vi "UHR-Fleezers Control (host) - 12.1.vi"() -> ()   [LabVIEW 2012] (continued)
            n1097 = Divide(x=w2495, y=w2493) -> (x/y=w2492:dbl[])
            n1098 = Divide(x=w2542, y=w2540) -> (x/y=w2526:dbl[])
            n1099 = Divide(x=w2541, y=w2540) -> (x/y=w2525:dbl[])
            n1100 = Divide(x=w2539, y=w2537) -> (x/y=w2524:dbl[])
            n1101 = Divide(x=w2538, y=w2537) -> (x/y=w2523:dbl[])
            n1102 = Divide(x=w2509, y=w2493) -> (x/y=w2508:dbl[])
            n1103 = Divide(x=w2507, y=w2491) -> (x/y=w2506:dbl[])
            n1104 = Build Array(w2526, w2525, w2540, w2524, w2523, w2537, w2492, w2508, w2493, w2490, w2506, w2491, w2504, w2503) -> (w2502:dbl[][])
            n1105 = Bundle("T1 Y", "T1 X", "T1 Sum", "T2 Y", "T2 X", "T2 Sum", "T1 FB Y", "T1 FB X", "T1 FB Sum", "T2 FB Y", "T2 FB X", "T2 FB Sum", "PSD X", "PSD Y Sum") -> (w2489:T39)  [unwired: 1 out]
            n1106 = To Word Integer(number=w2544) -> (16bit integer=w2488:i16[])
            n1107 = Cluster To Array(cluster=w2489) -> (array=w2535:string[])
          }
        }
      }
    }
    "AI labels" <- w1629
    n1108 = Decimate 1D Array(w1603) -> (w1627:u32[], w1571:u32[])
    n1109 = local read "DMA Update Period (s)"() -> (w1639:dbl)
    n1110 = Build Array(w1627, w1571) -> (w1697:u32[][])
    n1111 = local read "Data Period (s)"() -> (w1477:dbl)
    n1112 = local read "BD 1 Frequency 2 (MHz)"() -> (w1510:dbl)
    n1113 = local read "BD 1 Frequency 1 (MHz)"() -> (w1511:dbl)
    n1114 = Decimate 1D Array(w1518) -> (w1542:i16[], w1541:i16[], w1539:i16[], w1538:i16[])  [unwired: 9 out]
    n1115 = To Double Precision Float(number=w1697) -> (double precision float=w1698:dbl[][])
    n1116 = local read "APD Integration Time (s)"() -> (w1584:dbl)
    n1117 = Multiply(x=w1477, y="Trap Pos. Disp. Downsample") -> (x*y=w1475:dbl)
    n1118 = Divide(x=w1542, y=w1541) -> (x/y=w1543:dbl[])
    n1119 = Divide(x=w1539, y=w1538) -> (x/y=w1540:dbl[])
    n1120 = feedback #6(0.0) -> (w1556:dbl)
    n1121 = Add(x=w1639, y=w1556) -> (x+y=w1737:dbl)
    n1122 = feedback-in #6(w1737) -> ()
    n1123 = local read "AOM X Cal (nm/MHz)"() -> (w1508:dbl)
    n1124 = To Time Stamp(1:w1556) -> (0:w1555:timestamp)
    n1125 = Split 1D Array(array=w1543, index="N El. to Ave.") -> (second subarray=w1546:dbl[])  [unwired: 1 out]
    n1126 = Split 1D Array(array=w1540, index="N El. to Ave.") -> (second subarray=w1545:dbl[])  [unwired: 1 out]
    n1127 = Multiply(x=w1477, y="Trap Disp. Downsample") -> (x*y=w1557:dbl)
    "Display Period (s)" <- w1557
    n1128 = for "Trap AI" {
      tunnel: [w2287] -> w1731 mode=indexing
      tunnel: w1555 -> [w2277]
      tunnel: "Trap Disp. Downsample" -> [w2285]
      tunnel: w1630 -> [w2283] mode=indexing
      tunnel: w1477 -> [w2282]
      tunnel: w1629 -> [w2281] mode=indexing
      tunnel: w1554 -> [w2280]
      tunnel: [w2279] -> w1595 mode=indexing
      tunnel: w1557 -> [w2278]
      workers-P: _ -> [_]
      n1129 = Bundle By Name("Y"=w2283, "dt"=w2282) -> (w2284:waveform(dbl))  [unwired: 1 out]
      n1130 = Set Waveform Attribute(5:w2281, 6:w2280, 7:w2284) -> (3:w2279:waveform(dbl))  [unwired: 1 in, 2 out]
      n1131 = call "downsample 1D array - double.vi"("Ave N"=w2285, "Array In"=w2283) -> ("Array Out"=w2286:dbl[])  [unwired: 1 out]
      n1132 = Bundle By Name(cluster=w2279, "t0"=w2277, "Y"=w2286, "dt"=w2278) -> (w2287:waveform(dbl))
    }
    n1133 = Bundle("BD 1 Frequency 1 (MHz)"=w1511, "BD 1 Frequency 2 (MHz)"=w1510) -> (w1512:T40)  [unwired: 1 out]
    n1134 = call-poly <vilib>:"Mean.vi"("X"=w1545) -> ("mean"=w1533:dbl)  [unwired: 1 out]
    n1135 = call-poly <vilib>:"Mean.vi"("X"=w1546) -> ("mean"=w1534:dbl)  [unwired: 1 out]
    n1136 = Reciprocal(x=w1557) -> (1/x=→"Trap Disp. Freq. (Hz)":dbl)
    n1137 = Cluster To Array(cluster=w1512) -> (array=w1509:dbl[])
    n1138 = local read "Trap X AI1 (DMA)"() -> (w1544:T13)
    n1139 = local read "Data points/scans (MCL)"() -> (w1709:dbl)
    n1140 = To Fixed-Point(number=w1533) -> (fixed-point=w1531:fxp<+/-,16,1>)  [unwired: 1 in]
    n1141 = To Fixed-Point(number=w1534) -> (fixed-point=w1532:fxp<+/-,16,1>)  [unwired: 1 in]
    n1142 = Bundle("Trap 1 Pos.", "Trap 2 Pos.") -> (w1553:cluster{string, string})  [unwired: 1 out]
    n1143 = Bundle By Name(cluster=w1544, "Set 1"=w1532, "Set 2"=w1531) -> (→"Trap X AI1 (DMA)":T13)
    n1144 = Cluster To Array(cluster=w1553) -> (array=w1550:string[])
    n1145 = Bundle("APD 1", "APD 2") -> (w1730:cluster{string, string})  [unwired: 1 out]
    n1146 = Select(t=-1.0, s="Negate Y Axis", f=1.0) -> (s? t:f=w1494:dbl)
    n1147 = for "Trap Position" {
      tunnel: w1559 -> [w1926] mode=indexing
      tunnel: "Trap Pos. Disp. Downsample" -> [w1925]
      tunnel: w1475 -> [w1923]
      tunnel: w1555 -> [w1922]
      tunnel: w1554 -> [w1920]
      tunnel: w1550 -> [w1919] mode=indexing
      tunnel: [w1918] -> w1464 mode=indexing
      tunnel: w1509 -> [w1916] mode=indexing
      tunnel: w1508 -> [w1914]
      tunnel: w1494 -> [w1913]
      n1148 = call "downsample 1D array - double.vi"("Ave N"=w1925, "Array In"=w1926) -> ("Array Out"=w1924:dbl[])  [unwired: 1 out]
      n1149 = Subtract(x=w1924, y=w1916) -> (x-y=w1917:dbl[])
      n1150 = Multiply(x=w1914, y=w1917) -> (x*y=w1915:dbl[])
      n1151 = Multiply(x=w1913, y=w1915) -> (x*y=w1912:dbl[])
      n1152 = Bundle By Name("Y"=w1912, "dt"=w1923, "t0"=w1922) -> (w1921:waveform(dbl))  [unwired: 1 out]
      n1153 = Set Waveform Attribute(5:w1919, 6:w1920, 7:w1921) -> (3:w1918:waveform(dbl))  [unwired: 1 in, 2 out]
    }
    n1154 = Cluster To Array(cluster=w1730) -> (array=w1727:string[])
    n1155 = for "APD" {
      tunnel: w1698 -> [w2266] mode=indexing
      tunnel: w1584 -> [w2274]
      tunnel: [w2270] -> w1591 mode=indexing
      tunnel: "APD Disp. Scale" -> [w2271]
      tunnel: w1554 -> [w2269]
      tunnel: w1727 -> [w2268] mode=indexing
      tunnel: "APD Disp. Downsample" -> [w2264]
      tunnel: [w2267] -> w1726
      workers-P: _ -> [_]
      tunnel: w1555 -> [w2263]
      n1156 = call "integrate 1D array interval - double.vi"("Ave N"=w2264, "Array In"=w2266) -> ("Array Out"=w2265:dbl[])  [unwired: 1 out]
      n1157 = Multiply(x=w2274, y=w2264) -> (x*y=w2267:dbl)
      n1158 = Divide(x=w2265, y=w2271) -> (x/y=w2272:dbl[])
      n1159 = Bundle By Name("t0"=w2263, "Y"=w2272, "dt"=w2267) -> (w2273:waveform(dbl))  [unwired: 1 out]
      n1160 = Set Waveform Attribute(5:w2268, 6:w2269, 7:w2273) -> (3:w2270:waveform(dbl))  [unwired: 1 in, 2 out]
    }
    "APD Display Period (s)" <- w1726
    n1161 = Reciprocal(x=w1726) -> (1/x=→"APD Display Freq. (Hz)":dbl)
    n1162 = local read "Display Period (s)"() -> (w1615:dbl)
    n1163 = Increment(x=w1709) -> (x+1=w1710:dbl)
    n1164 = To Double Precision Float(number=w1627) -> (double precision float=w1626:dbl[])
    n1165 = Index Array(array=w1464, index=0) -> (element=w1468:waveform(dbl))
    n1166 = Index Array(array=w1464, index=1) -> (element=w1463:waveform(dbl))
    n1167 = feedback #7(w1710) -> (w1713:dbl)
    n1168 = Select(t=0, s=w1700, f=w1713) -> (s? t:f=w1706:dbl)
    n1169 = Array Size(array=w1626) -> (size(s)=w1712:i32)
    n1170 = Add(x=w1712, y=w1706) -> (x+y=w1707:dbl)
    n1171 = Unbundle By Name(w1468) -> ("Y"=w1469:dbl[])
    n1172 = feedback #8(w1627) -> (w1696:u32[])
    n1173 = Build Array (concatenate)(w1696, w1627) -> (w1693:u32[])
    n1174 = feedback #9(w1571) -> (w1590:u32[])
    n1175 = Divide(x="Bead Sep. Int. Time (s)", y=w1615) -> (x/y=w1504:dbl)
    n1176 = Build Array (concatenate)(w1590, w1571) -> (w1589:u32[])
    n1177 = Add(x=w1469, y="FB Trap Pos Offset") -> (x+y=w1467:dbl[])
    "T1 x pos data" <- w1467
    n1178 = Greater?(x=w1707, y=w1709) -> (0:w1708:bool)
    n1179 = feedback #10(w1467) -> (w1506:dbl[])
    n1180 = Build Array (concatenate)(w1467, w1506) -> (w1505:dbl[])
    n1181 = Bundle By Name(cluster=w1468, "Y"=w1467) -> (w1466:waveform(dbl))
    n1182 = Select(t=w1706, s=w1708, f=w1707) -> (s? t:f=w1705:dbl)
    n1183 = feedback-in #7(w1705) -> ()
    n1184 = Array Size(array=w1693) -> (size(s)=w1690:i32)
    n1185 = Array Size(array=w1627) -> (size(s)=w1692:i32)
    n1186 = local read "MCL Scanning"() -> (w1703:bool)
    n1187 = local read "APD Integration Time (s)"() -> (w1598:dbl)
    n1188 = Bundle(w1466, w1463) -> (w1462:cluster{waveform(dbl), waveform(dbl)})  [unwired: 1 out]
    n1189 = Build Array (concatenate)(w1591, w1731) -> (w1593:waveform(dbl)[])
    "All Signals" <- w1593
    n1190 = Split 1D Array(array=w1505, index=w1504) -> (first subarray=w1498:dbl[])  [unwired: 1 out]
    n1191 = feedback-in #10(w1498) -> ()
    n1192 = Multiply(x=w1692, y="APD Ave N") -> (x*y=w1691:dbl)
    n1193 = Greater?(x=w1690, y=w1691) -> (0:w1694:bool)
    n1194 = Not(x=w1708) -> (.not. x?=w1702:bool)
    n1195 = Cluster To Array(cluster=w1462) -> (array=w1438:waveform(dbl)[])
    "Trap Positions" <- w1438
    n1196 = To Double Precision Float(number=w1571) -> (double precision float=w1570:dbl[])
    n1197 = call-poly <vilib>:"Mean.vi"("X"=w1498) -> ("mean"=w1497:dbl)  [unwired: 1 out]
    "Mean T1 Position (nm)" <- w1497
    n1198 = Subtract(x=w1498, y=w1497) -> (x-y=w1503:dbl[])
    n1199 = Square(x=w1503) -> (x^2=w1502:dbl[])
    n1200 = And(x=w1702, y=w1703) -> (x .and. y?=w1704:bool)
    n1201 = call-poly <vilib>:"Mean.vi"("X"=w1502) -> ("mean"=w1501:dbl)  [unwired: 1 out]
    n1202 = case shown="True" w1694 {
      tunnel: w1693 -> [w2046 w2053]
      tunnel: [w2046 w2051] -> w1644
      tunnel: w1691 -> [_ w2048]
      tunnel: w1690 -> [_ w2052]
      tunnel: w1589 -> [w2045 w2050]
      tunnel: [w2045 w2047] -> w1586
      frame False {
      }
      frame True {
        n1203 = Subtract(x=w2052, y=w2048) -> (x-y=w2049:dbl)
        n1204 = Array Subset(array=w2053, index=w2049, length=w2048) -> (w2051:u32[])
        n1205 = Array Subset(array=w2050, index=w2049, length=w2048) -> (w2047:u32[])
      }
    }
    n1206 = feedback-in #8(w1644) -> ()
    n1207 = feedback-in #9(w1586) -> ()
    n1208 = Square Root(x=w1501) -> (sqrt(x)=w1500:dbl)
    n1209 = Or(x=w1704, y=w1700) -> (x .or. y?=w1701:bool)
    n1210 = Equal?(x="Tab Control 6", y=T28."High Res Display") -> (x = y?=w1633:bool)
    n1211 = Multiply(x="APD Disp. Scale", y=w1591) -> (x*y=w1600:waveform(dbl)[])
    n1212 = Multiply(x=10.0, y=w1500) -> (x*y=→"Trap 1 Position RMS (A)":dbl)
    n1213 = Multiply(x="APD Disp. Downsample", y=w1598) -> (x*y=w1596:dbl)
    n1214 = Divide(x=w1600, y=w1596) -> (x/y=w1568:waveform(dbl)[])
    n1215 = case "For displaying the high resolution display (no downsampling)" shown="True" w1633 {
      tunnel: w1595 -> [_ w1946]
      frame False {
      }
      frame True {
        n1216 = Index Array(array=w1946, index="High Res. Display") -> (element=w1947:waveform(dbl))
        n1217 = call <vilib>:"Std Deviation and Variance.vi"("X"=w1947) -> ("mean"=w1954:dbl, "standard deviation"=w1959:dbl)  [unwired: 1 in, 1 out]
        "Mean Intensity" <- w1954
        "Sigma" <- w1959
        n1218 = Subtract(x=w1947, y=w1954) -> (x-y=w1953:waveform(dbl))
        n1219 = Select(t=w1953, s="Subtract mean", f=w1947) -> (s? t:f=→"1 Channel":waveform(dbl))
        n1220 = Divide(x=w1959, y=w1954) -> (x/y=→"Sigma/Mean":dbl)
        n1221 = feedback #11(1) -> (w1948:i32)
        n1222 = Greater Or Equal?(x=w1948, y="Slow mean N ave.") -> (x >= y?=w1961:bool)
        n1223 = Increment(x=w1948) -> (x+1=w1963:i32)
        n1224 = Select(t=1, s=w1961, f=w1963) -> (s? t:f=w1950:i32)
        n1225 = feedback-in #11(w1950) -> ()
        n1226 = feedback #12() -> (w1951:waveform(dbl))  [unwired: 1 out]
        n1227 = case shown="Default" w1948 {
          tunnel: [w1966 w1969] -> w1952
          tunnel: w1951 -> [w1968 _]
          tunnel: w1947 -> [w1967 w1969]
          frame Default {
            n1228 = call-poly <vilib>:"Append Waveforms.vi"("waveform B"=w1967, "waveform A"=w1968) -> ("waveform out"=w1966:waveform(dbl))  [unwired: 1 in, 8 out]
          }
          frame 1 {
          }
        }
        n1229 = feedback-in #12(w1952) -> ()
        n1230 = case shown="True" w1961 {
          tunnel: w1952 -> [_ w1965]
          frame False {
          }
          frame True {
            n1231 = call-poly <vilib>:"Mean.vi"("X"=w1965) -> ("mean"=→"Slow mean":dbl)  [unwired: 1 out]
          }
        }
      }
    }
    n1232 = Index Array(array=w1568, index=0) -> (element=w1578:waveform(dbl))
    n1233 = Index Array(array=w1568, index=1) -> (element=w1576:waveform(dbl))
    n1234 = case "For computing FFTs for display" shown="True" "Compute FFT" {
      tunnel: w1595 -> [_ w2660]
      frame False {
      }
      frame True {
        n1235 = Build Array("FFT 1 Choice 1", "FFT 1 Choice 2", "FFT 2 Choice 1", "FFT 2 Choice 2") -> (w2653:u16[])
        n1236 = Array Size(array=w2660) -> (size(s)=w2659:i32)
        n1237 = feedback-in #13(w2653) -> ()
        n1238 = feedback #13(u16[] [100, 100, 100, 100]) -> (w2654:u16[])
        n1239 = feedback-in #14("# Spectra to Ave.") -> ()
        n1240 = feedback #14("# Spectra to Ave.") -> (w2651:dbl)
        n1241 = Not Equal?(x="# Spectra to Ave.", y=w2651) -> (x != y?=w2650:bool)
        n1242 = Not Equal?(x=w2653, y=w2654) -> (x != y?=w2652:bool)
        n1243 = feedback #15(1.0) -> (w2637:dbl)
        n1244 = Compound Arithmetic op=OR("Reset FFT", w2652, w2650) -> (w2635:bool)
        n1245 = Select(t=1.0, s=w2635, f=w2637) -> (s? t:f=w2639:dbl)
        n1246 = Greater?(x=w2639, y="# Spectra to Ave.") -> (0:w2658:bool)
        n1247 = Increment(x=w2639) -> (x+1=w2638:dbl)
        n1248 = feedback-in #15(w2638) -> ()
        n1249 = local read "DMA Update Period (s)"() -> (w2633:dbl)
        n1250 = Multiply(x="# Spectra to Ave.", y=w2633) -> (x*y=→"Ave. Time (s)":dbl)
        n1251 = Build Array(cluster{"f0":dbl, "df":dbl, "magnitude":dbl[]} {"f0"=0.0, "df"=0.0, "magnitude"=[]} ("PSD")) -> (w2642:cluster{"f0":dbl, "df":dbl, "magnitude":dbl[]}[])
        n1252 = Build Array(w2642, w2642, w2642, w2642) -> (w2644:T41)
        n1253 = feedback #16(w2644) -> (w2649:T41)
        n1254 = for {
          N: 4 -> [_]
          tunnel: w2653 -> [w2682] mode=indexing
          tunnel: w2660 -> [w2683]
          tunnel: w2659 -> [w2685]
          tunnel: w2635 -> [w2678]
          tunnel: w2658 -> [w2677]
          tunnel: "# Spectra to Ave." -> [w2676]
          tunnel: [w2675] -> w2648 mode=indexing
          tunnel: w2649 -> [w2680] mode=indexing
          tunnel: [w2679] -> w2636 mode=indexing
          tunnel: w2639 -> [w2674]
          n1255 = Less?(x=w2682, y=w2685) -> (x < y?=w2684:bool)
          n1256 = Index Array(array=w2683, index=w2682) -> (element=w2681:waveform(dbl))
          n1257 = case shown="True" w2684 {
            tunnel: w2681 -> [_ w2702]
            tunnel: w2680 -> [w2687 w2700]
            tunnel: [w2687 w2688] -> w2679
            tunnel: w2678 -> [_ w2699]
            tunnel: w2677 -> [_ w2692]
            tunnel: w2676 -> [_ w2691]
            tunnel: [cluster{"f0":dbl, "df":dbl, "magnitude":dbl[]} {"f0"=0.0, "df"=0.0, "magnitude"=[]} ("PSD") w2693] -> w2675
            tunnel: w2674 -> [_ w2690]
            frame False {
            }
            frame True {
              n1258 = call <vilib>:"Std Deviation and Variance.vi"("X"=w2702) -> ("mean"=w2703:dbl)  [unwired: 1 in, 2 out]
              n1259 = Subtract(x=w2702, y=w2703) -> (x-y=w2701:waveform(dbl))
              n1260 = xnode "Spectral Measurements"("Signals"=w2701) -> ("PSD"=w2695:cluster{"f0":dbl, "df":dbl, "magnitude":dbl[]})  [unwired: 1 in, 1 out]
              n1261 = case shown="False" w2699 {
                tunnel: w2700 -> [w2712 _]
                tunnel: [w2708 w2717] -> w2688
                tunnel: w2695 -> [w2711 w2718]
                tunnel: w2692 -> [w2710 _]
                frame False {
                  n1262 = Build Array (concatenate)(w2712, w2711) -> (w2709:cluster{"f0":dbl, "df":dbl, "magnitude":dbl[]}[])
                  n1263 = case shown="True" w2710 {
                    tunnel: w2709 -> [w2713 w2716]
                    tunnel: [w2713 w2714] -> w2708
                    frame False {
                    }
                    frame True {
                      n1264 = Delete From Array(array=w2716, index=0) -> (array with subset deleted=w2714:cluster{"f0":dbl, "df":dbl, "magnitude":dbl[]}[])  [unwired: 1 in, 1 out]
                    }
                  }
                }
                frame True {
                  n1265 = Build Array(w2718) -> (w2717:cluster{"f0":dbl, "df":dbl, "magnitude":dbl[]}[])
                }
              }
              n1266 = for {
                tunnel: w2688 -> [w2707] mode=indexing
                tunnel: [w2706] -> w2698 mode=indexing
                workers-P: _ -> [_]
                n1267 = Unbundle By Name(w2707) -> ("magnitude"=w2706:dbl[])
              }
              n1268 = Transpose 2D Array(2D array=w2698) -> (transposed array=w2697:dbl[][])
              n1269 = for {
                tunnel: w2697 -> [w2705] mode=indexing
                tunnel: [w2704] -> w2696 mode=indexing
                workers-P: _ -> [_]
                n1270 = Add Array Elements(numeric array=w2705) -> (sum=w2704:dbl)
              }
              n1271 = Select(t=w2691, s=w2692, f=w2690) -> (s? t:f=w2689:dbl)
              n1272 = Divide(x=w2696, y=w2689) -> (x/y=w2694:dbl[])
              n1273 = Bundle By Name(cluster=w2695, "magnitude"=w2694) -> (w2693:cluster{"f0":dbl, "df":dbl, "magnitude":dbl[]})
            }
          }
        }
        n1274 = case shown="True" w2635 {
          tunnel: w2636 -> [w2667 w2673]
          tunnel: [w2667 w2668] -> w2634
          frame False {
          }
          frame True {
            n1275 = Array Subset(array=w2673, index (row)=0 ("index"), length (row)=4 ("length"), index (col)=0 ("index"), length (col)=1 ("length")) -> (w2668:T41)
          }
        }
        n1276 = feedback-in #16(w2634) -> ()
        n1277 = Split 1D Array(array=w2648, index=2) -> (first subarray=→"FFT 1":cluster{"f0":dbl, "df":dbl, "magnitude":dbl[]}[], second subarray=→"FFT 2":cluster{"f0":dbl, "df":dbl, "magnitude":dbl[]}[])
      }
    }
    n1278 = case "For plotting results of scanning MCL" shown="True" w1701 {
      tunnel: w1700 -> [_ w2086]
      tunnel: w1626 -> [_ w2182]
      tunnel: w1709 -> [_ _]
      tunnel: w1595 -> [_ w2156]
      tunnel: w1570 -> [_ w2087]
      tunnel: w1569 -> [_ w2060]
      frame False {
      }
      frame True {
        w2067 = u32 0 items=["Horizontal", "Vertical", "Central", "1st Diagonal", "2nd Diagonal"] ("Type of Symmetry")
        w2095 = u32 0 items=["Horizontal", "Vertical", "Central", "1st Diagonal", "2nd Diagonal"] ("Type of Symmetry")
        w2098 = u32 0 items=["Horizontal", "Vertical", "Central", "1st Diagonal", "2nd Diagonal"] ("Type of Symmetry")
        w2127 = u32 0 items=["Horizontal", "Vertical", "Central", "1st Diagonal", "2nd Diagonal"] ("Type of Symmetry")
        n1279 = Index Array(array=w2156, index=10) -> (element=w2162:waveform(dbl))
        n1280 = Index Array(array=w2156, index=11) -> (element=w2159:waveform(dbl))
        n1281 = local read "Cycles/step (MCL)"() -> (w2112:u64)
        n1282 = Index Array(array=w2156, index="Channel") -> (element=w2158:waveform(dbl))
        n1283 = Unbundle(w2060) -> ("New Image"=w2059:T2, "New Image"=w2058:T2, "New Image"=w2057:T2, "New Image"=w2056:T2)
        n1284 = Unbundle By Name(w2162) -> ("Y"=w2114:dbl[])
        n1285 = Unbundle By Name(w2159) -> ("Y"=w2116:dbl[])
        n1286 = Unbundle By Name(w2158) -> ("Y"=w2121:dbl[])
        n1287 = call "downsample 1D array - double.vi"("Ave N"=w2112, "Array In"=w2114) -> ("Array Out"=w2113:dbl[])  [unwired: 1 out]
        n1288 = call "downsample 1D array - double.vi"("Ave N"=w2112, "Array In"=w2116) -> ("Array Out"=w2115:dbl[])  [unwired: 1 out]
        n1289 = call "downsample 1D array - double.vi"("Ave N"=w2112, "Array In"=w2121) -> ("Array Out"=w2120:dbl[])  [unwired: 1 out]
        n1290 = feedback #17(w2182) -> (w2183:dbl[])
        n1291 = Build Array (concatenate)(w2183, w2182) -> (w2164:dbl[])
        n1292 = feedback #18(w2087) -> (w2089:dbl[])
        n1293 = Build Array (concatenate)(w2089, w2087) -> (w2088:dbl[])
        n1294 = local read "Scan steps (MCL)"() -> (w2069:u64)
        n1295 = Select(t=w2182, s=w2086, f=w2164) -> (s? t:f=w2168:dbl[])
        n1296 = feedback-in #17(w2168) -> ()
        n1297 = Select(t=w2087, s=w2086, f=w2088) -> (s? t:f=w2070:dbl[])
        n1298 = feedback-in #18(w2070) -> ()
        n1299 = local read "Scan lines (y)"() -> (w2055:u64)
        n1300 = local read "N APD Samp/step"() -> (w2071:dbl)
        n1301 = feedback #19(w2113) -> (w2170:dbl[])
        n1302 = Build Array (concatenate)(w2170, w2113) -> (w2161:dbl[])
        n1303 = feedback #20(w2120) -> (w2180:dbl[])
        n1304 = Build Array (concatenate)(w2180, w2120) -> (w2179:dbl[])
        n1305 = feedback #21(w2115) -> (w2172:dbl[])
        n1306 = Build Array (concatenate)(w2172, w2115) -> (w2173:dbl[])
        n1307 = Select(t=w2113, s=w2086, f=w2161) -> (s? t:f=w2117:dbl[])
        n1308 = feedback-in #19(w2117) -> ()
        n1309 = Select(t=w2120, s=w2086, f=w2179) -> (s? t:f=w2119:dbl[])
        n1310 = feedback-in #20(w2119) -> ()
        n1311 = Select(t=w2115, s=w2086, f=w2173) -> (s? t:f=w2118:dbl[])
        n1312 = feedback-in #21(w2118) -> ()
        n1313 = Multiply(x=w2069, y=u64 2) -> (x*y=w2054:u64)
        n1314 = call "integrate 1D array interval - double.vi"("Ave N"=w2071, "Array In"=w2070) -> ("Array Out"=w2082:dbl[])  [unwired: 1 out]
        n1315 = call "integrate 1D array interval - double.vi"("Ave N"=w2071, "Array In"=w2168) -> ("Array Out"=w2167:dbl[])  [unwired: 1 out]
        n1316 = Array Size(array=w2082) -> (size(s)=w2083:i32)
        n1317 = Array Size(array=w2167) -> (size(s)=w2169:i32)
        n1318 = Multiply(x=w2055, y=w2054) -> (x*y=w2085:u64)
        n1319 = Multiply(x=w2055, y=w2054) -> (x*y=w2177:u64)
        n1320 = call-poly <vilib>:"Mean.vi"("X"=w2117) -> ("mean"=w2101:dbl)  [unwired: 1 out]
        n1321 = Subtract(x=w2085, y=w2083) -> (x-y=w2076:u64)
        n1322 = call-poly <vilib>:"Mean.vi"("X"=w2119) -> ("mean"=w2106:dbl)  [unwired: 1 out]
        n1323 = call-poly <vilib>:"Mean.vi"("X"=w2118) -> ("mean"=w2104:dbl)  [unwired: 1 out]
        n1324 = call-poly <vilib>:"Mean.vi"("X"=w2082) -> ("mean"=w2073:dbl)  [unwired: 1 out]
        n1325 = Subtract(x=w2177, y=w2169) -> (x-y=w2111:u64)
        n1326 = call-poly <vilib>:"Mean.vi"("X"=w2167) -> ("mean"=w2108:dbl)  [unwired: 1 out]
        n1327 = Initialize Array(1.0 ("element"), w2076) -> (w2072:dbl[])
        n1328 = Initialize Array(1.0 ("element"), w2111) -> (w2102:dbl[])
        n1329 = Multiply(x=w2072, y=w2073) -> (x*y=w2074:dbl[])
        n1330 = Multiply(x=w2102, y=w2104) -> (x*y=w2105:dbl[])
        n1331 = Multiply(x=w2102, y=w2106) -> (x*y=w2107:dbl[])
        n1332 = Multiply(x=w2102, y=w2101) -> (x*y=w2103:dbl[])
        n1333 = Multiply(x=w2102, y=w2108) -> (x*y=w2109:dbl[])
        n1334 = Build Array (concatenate)(w2117, w2103) -> (w2171:dbl[])
        n1335 = Build Array (concatenate)(w2119, w2107) -> (w2175:dbl[])
        n1336 = Build Array (concatenate)(w2118, w2105) -> (w2174:dbl[])
        n1337 = Build Array (concatenate)(w2082, w2074) -> (w2084:dbl[])
        n1338 = Build Array (concatenate)(w2167, w2109) -> (w2176:dbl[])
        n1339 = Reshape Array(w2171, w2055, w2054) -> (w2137:dbl[][])
        n1340 = Reshape Array(w2084, w2055, w2054) -> (w2080:dbl[][])
        n1341 = Reshape Array(w2175, w2055, w2054) -> (w2129:dbl[][])
        n1342 = Reshape Array(w2174, w2055, w2054) -> (w2144:dbl[][])
        n1343 = Reshape Array(w2176, w2055, w2054) -> (w2154:dbl[][])
        n1344 = Array Subset(array=w2144, index (col)=0 ("index"), length (col)=w2069) -> (w2149:dbl[][])  [unwired: 2 in]
        n1345 = Array Subset(array=w2144, index (col)=w2069) -> (w2147:dbl[][])  [unwired: 3 in]
        n1346 = Array Subset(array=w2129, index (col)=0 ("index"), length (col)=w2069) -> (w2135:dbl[][])  [unwired: 2 in]
        n1347 = Array Subset(array=w2129, index (col)=w2069) -> (w2133:dbl[][])  [unwired: 3 in]
        n1348 = Array Subset(array=w2080, index (col)=0 ("index"), length (col)=w2069) -> (w2079:dbl[][])  [unwired: 2 in]
        n1349 = Array Subset(array=w2080, index (col)=w2069) -> (w2077:dbl[][])  [unwired: 3 in]
        n1350 = Array Subset(array=w2154, index (col)=0 ("index"), length (col)=w2069) -> (w2153:dbl[][])  [unwired: 2 in]
        n1351 = Array Subset(array=w2154, index (col)=w2069) -> (w2151:dbl[][])  [unwired: 3 in]
        n1352 = Array Subset(array=w2137, index (col)=0 ("index"), length (col)=w2069) -> (w2142:dbl[][])  [unwired: 2 in]
        n1353 = Array Subset(array=w2137, index (col)=w2069) -> (w2140:dbl[][])  [unwired: 3 in]
        n1354 = for {
          tunnel: w2149 -> [w2191] mode=indexing
          tunnel: [w2190] -> w2148 mode=indexing
          workers-P: _ -> [_]
          n1355 = Reverse 1D Array(array=w2191) -> (reversed array=w2190:dbl[])
        }
        n1356 = for {
          tunnel: w2135 -> [w2187] mode=indexing
          tunnel: [w2186] -> w2134 mode=indexing
          workers-P: _ -> [_]
          n1357 = Reverse 1D Array(array=w2187) -> (reversed array=w2186:dbl[])
        }
        n1358 = for {
          tunnel: w2079 -> [w2185] mode=indexing
          tunnel: [w2184] -> w2078 mode=indexing
          workers-P: _ -> [_]
          n1359 = Reverse 1D Array(array=w2185) -> (reversed array=w2184:dbl[])
        }
        n1360 = for {
          tunnel: w2153 -> [w2193] mode=indexing
          tunnel: [w2192] -> w2152 mode=indexing
          workers-P: _ -> [_]
          n1361 = Reverse 1D Array(array=w2193) -> (reversed array=w2192:dbl[])
        }
        n1362 = for {
          tunnel: w2142 -> [w2189] mode=indexing
          tunnel: [w2188] -> w2141 mode=indexing
          workers-P: _ -> [_]
          n1363 = Reverse 1D Array(array=w2189) -> (reversed array=w2188:dbl[])
        }
        n1364 = Index Array(array=w2154, index (row)=0) -> (element=→"Waveform Graph":dbl[])  [unwired: 1 in]
        n1365 = Add(x=w2148, y=w2147) -> (x+y=w2146:dbl[][])
        n1366 = Add(x=w2134, y=w2133) -> (x+y=w2132:dbl[][])
        n1367 = Add(x=w2078, y=w2077) -> (x+y=w2062:dbl[][])
        n1368 = Add(x=w2152, y=w2151) -> (x+y=w2126:dbl[][])
        n1369 = Add(x=w2141, y=w2140) -> (x+y=w2139:dbl[][])
        n1370 = Divide(x=w2132, y=2) -> (x/y=w2130:dbl[][])
        n1371 = Divide(x=w2146, y=2) -> (x/y=w2091:dbl[][])
        n1372 = Divide(x=w2139, y=2) -> (x/y=w2093:dbl[][])
        n1373 = To Single Precision Float(number=w2126) -> (single precision float=w2125:sgl[][])
        n1374 = Transpose 2D Array(2D array=w2130) -> (transposed array=→"Data map":dbl[][])
        n1375 = To Single Precision Float(number=w2062) -> (single precision float=w2066:sgl[][])
        n1376 = To Single Precision Float(number=w2091) -> (single precision float=w2097:sgl[][])
        n1377 = To Single Precision Float(number=w2093) -> (single precision float=w2094:sgl[][])
        n1378 = call "IMAQ ArrayToImage"("Image Pixels (Float)"=w2125, "Image"=w2059) -> ("Image Out"=w2128:T2)  [unwired: 8 in, 1 out]
        n1379 = call "IMAQ ArrayToImage"("Image Pixels (Float)"=w2066, "Image"=w2058) -> ("Image Out"=w2068:T2)  [unwired: 8 in, 1 out]
        n1380 = call "IMAQ ArrayToImage"("Image Pixels (Float)"=w2097, "Image"=w2057) -> ("Image Out"=w2099:T2)  [unwired: 8 in, 1 out]
        n1381 = call "IMAQ ArrayToImage"("Image Pixels (Float)"=w2094, "Image"=w2056) -> ("Image Out"=w2096:T2)  [unwired: 8 in, 1 out]
        n1382 = call "IMAQ Symmetry"("Type of Symmetry"=w2127, "Image Src"=w2128) -> ("Image Dst Out"=w2123:T2)  [unwired: 3 in, 1 out]
        n1383 = call "IMAQ Symmetry"("Type of Symmetry"=w2067, "Image Src"=w2068) -> ("Image Dst Out"=w2064:T2)  [unwired: 3 in, 1 out]
        n1384 = call "IMAQ Symmetry"("Type of Symmetry"=w2098, "Image Src"=w2099) -> ("Image Dst Out"=→"Detection Laser X":T2)  [unwired: 3 in, 1 out]
        n1385 = call "IMAQ Symmetry"("Type of Symmetry"=w2095, "Image Src"=w2096) -> ("Image Dst Out"=→"Detection Laser Y":T2)  [unwired: 3 in, 1 out]
        n1386 = call "IMAQ Set Simple Calibration"("Calibration Axis Info"=T29 {"Origin Pixel"={"X"=0.0, "Y"=0.0}, "Angle Relative to Horizontal (deg)"=0.0, "Axis Reference"=0}, "Grid Descriptor"=T30 {"X Step"=0.3, "Y Step"=0.3, "Unit"=enum."Undefined"}, "Image"=w2123) -> ("Calibrated Image"=→"APD 1":T2)  [unwired: 7 in, 1 out]
        n1387 = call "IMAQ Set Simple Calibration"("Calibration Axis Info"=T29 {"Origin Pixel"={"X"=0.0, "Y"=0.0}, "Angle Relative to Horizontal (deg)"=0.0, "Axis Reference"=0}, "Grid Descriptor"=T30 {"X Step"=0.3, "Y Step"=0.3, "Unit"=enum."Undefined"}, "Image"=w2064) -> ("Calibrated Image"=→"APD 2":T2)  [unwired: 7 in, 1 out]
      }
    }
    n1388 = Subtract(x=w1576, y="APD 2 Offset") -> (x-y=w1573:waveform(dbl))
    n1389 = Subtract(x=w1578, y="APD 1 Offset") -> (x-y=w1574:waveform(dbl))
    n1390 = Index Array(array=w1593, index=3) -> (element=w1653:waveform(dbl))
    n1391 = Index Array(array=w1593, index=6) -> (element=w1650:waveform(dbl))
    n1392 = Build Array(w1574, w1573) -> (→"APD Chart":waveform(dbl)[])
    n1393 = Array Size(array=w1644) -> (size(s)=w1689:i32)
    n1394 = call <vilib>:"Std Deviation and Variance.vi"("X"=w1586) -> ("standard deviation"=w1585:dbl)  [unwired: 1 in, 2 out]
    n1395 = Add Array Elements(numeric array=w1586) -> (sum=w1588:u32)
    n1396 = Add Array Elements(numeric array=w1644) -> (sum=w1699:u32)
    n1397 = call <vilib>:"Std Deviation and Variance.vi"("X"=w1644) -> ("standard deviation"=w1643:dbl)  [unwired: 1 in, 2 out]
    n1398 = Divide(x="T1 offset_x (mV)", y=1000.0) -> (x/y=w1654:dbl)
    n1399 = Divide(x=w1585, y=w1584) -> (x/y=w1581:dbl)
    "Rate sigma (Hz) 2" <- w1581
    n1400 = Multiply(x=w1584, y=w1689) -> (x*y=w1587:dbl)
    "Int. Time (s)" <- w1587
    n1401 = Divide(x=w1588, y=w1587) -> (x/y=w1582:dbl)
    "APD 2 Rate (Hz)" <- w1582
    n1402 = Divide(x=w1699, y=w1587) -> (x/y=w1641:dbl)
    "APD 1 Rate (Hz)" <- w1641
    n1403 = Divide(x=w1643, y=w1584) -> (x/y=w1642:dbl)
    "Rate sigma (Hz)" <- w1642
    n1404 = Divide(x=w1581, y=w1582) -> (x/y=→"Sigma/Mean 2":dbl)
    n1405 = Divide(x=w1642, y=w1641) -> (x/y=→"Sigma/Mean":dbl)
    n1406 = feedback-in #22("Calibration") -> ()
    n1407 = feedback #22(u16 1 ("Calibration")) -> (w1672:u16)
    n1408 = Divide(x="T2 offset_x (mV)", y=1000.0) -> (x/y=w1652:dbl)
    n1409 = case shown="0, Default" "Calibration" {
      tunnel: "T1 alpha_x (nm/V)" -> [_ w2022 w2043]
      tunnel: "T1 kappa_x (pN/nm)" -> [_ _ w2033]
      tunnel: "T2 alpha_x (nm/V)" -> [_ w2021 w2041]
      tunnel: "T2 kappa_x (pN/nm)" -> [_ _ w2034]
      tunnel: w1653 -> [w2004 w2019 w2039]
      tunnel: w1650 -> [w2003 w2017 w2037]
      tunnel: [w2004 w2016 w2036] -> w1681
      tunnel: [w2003 w2015 w2035] -> w1680
      tunnel: ["T1 X (V)" ("Label.Text") "T1 X (nm)" ("Label.Text") "T1 X (pN)" ("Label.Text")] -> w1669
      tunnel: ["T2 X (V)" ("Label.Text") "T2 X (nm)" ("Label.Text") "T2 X (pN)" ("Label.Text")] -> w1668
      tunnel: ["Position (V)" ("Label.Text") "Position (nm)" ("Label.Text") "Force (pN)" ("Label.Text")] -> w1670
      tunnel: w1652 -> [_ w2007 w2026]
      tunnel: w1654 -> [_ w2010 w2028]
      tunnel: ["Mean (V)" ("Label.Text") "Mean (nm)" ("Label.Text") "Mean (pN)" ("Label.Text")] -> w1665
      tunnel: ["Difference (V)" ("Label.Text") "Difference (nm)" ("Label.Text") "Difference (pN)" ("Label.Text")] -> w1601
      frame 0, Default {
      }
      frame 1 {
        n1410 = Unbundle By Name(w2019) -> ("Y"=w2023:dbl[])
        n1411 = Unbundle By Name(w2017) -> ("Y"=w2008:dbl[])
        n1412 = Subtract(x=w2023, y=w2010) -> (x-y=w2011:dbl[])
        n1413 = Subtract(x=w2008, y=w2007) -> (x-y=w2009:dbl[])
        n1414 = Multiply(x=w2009, y=w2021) -> (x*y=w2018:dbl[])
        n1415 = Multiply(x=w2022, y=w2011) -> (x*y=w2020:dbl[])
        n1416 = Bundle By Name(cluster=w2017, "Y"=w2018) -> (w2015:waveform(dbl))
        n1417 = Bundle By Name(cluster=w2019, "Y"=w2020) -> (w2016:waveform(dbl))
      }
      frame 2 {
        n1418 = Unbundle By Name(w2039) -> ("Y"=w2044:dbl[])
        n1419 = Unbundle By Name(w2037) -> ("Y"=w2042:dbl[])
        n1420 = Subtract(x=w2042, y=w2026) -> (x-y=w2027:dbl[])
        n1421 = Subtract(x=w2044, y=w2028) -> (x-y=w2029:dbl[])
        n1422 = Compound Arithmetic op=MULTIPLY(w2027, w2041, w2034) -> (w2038:dbl[])
        n1423 = Compound Arithmetic op=MULTIPLY(w2033, w2043, w2029) -> (w2040:dbl[])
        n1424 = Bundle By Name(cluster=w2037, "Y"=w2038) -> (w2035:waveform(dbl))
        n1425 = Bundle By Name(cluster=w2039, "Y"=w2040) -> (w2036:waveform(dbl))
      }
    }
    n1426 = Not Equal?(x=w1672, y="Calibration") -> (x != y?=w1631:bool)
    n1427 = case shown="True" w1631 {
      tunnel: w1670 -> [_ w1997]
      tunnel: w1669 -> [_ w1996]
      tunnel: w1668 -> [_ w1995]
      tunnel: w1665 -> [_ w1994]
      tunnel: w1601 -> [_ w1993]
      frame False {
      }
      frame True {
        n1428 = property on="Force" class="WFChart (strict)"("YScale.NameLbl.Text"=w1997) -> ()  [unwired: 2 in, 2 out]
        n1429 = property on="T2 X" class="DigNum (strict)"("Caption.Text"=w1995) -> ()  [unwired: 2 in, 2 out]
        n1430 = property on="T1 X" class="DigNum (strict)"("Caption.Text"=w1996) -> ()  [unwired: 2 in, 2 out]
        n1431 = property on="Mean" class="DigNum (strict)"("Caption.Text"=w1994) -> ()  [unwired: 2 in, 2 out]
        n1432 = property on="Difference" class="DigNum (strict)"("Caption.Text"=w1993) -> ()  [unwired: 2 in, 2 out]
      }
    }
    n1433 = Unbundle By Name(w1653) -> ("Y"=w1656:dbl[])
    n1434 = Unbundle By Name(w1650) -> ("Y"=w1659:dbl[])
    n1435 = Subtract(x=w1656, y=w1654) -> (x-y=w1657:dbl[])
    n1436 = Subtract(x=w1659, y=w1652) -> (x-y=w1658:dbl[])
    n1437 = Multiply(x=w1658, y="T2 alpha_x (nm/V)") -> (x*y=w1443:dbl[])
    n1438 = Multiply(x="T1 alpha_x (nm/V)", y=w1657) -> (x*y=w1444:dbl[])
    n1439 = Not(x="Trap Trig. Fl.") -> (.not. x?=w1480:bool)
    n1440 = Multiply(x=w1680, y=-1.0) -> (x*y=w1661:waveform(dbl))
    n1441 = Subtract(x=w1444, y=w1443) -> (x-y=w1649:dbl[])
    n1442 = Unbundle By Name(w1680) -> ("Y"=w1620:dbl[])
    n1443 = Unbundle By Name(w1681) -> ("Y"=w1445:dbl[])
    n1444 = Negate(x=w1649) -> (-x=w1441:dbl[])
    n1445 = Build Array(w1681, w1661) -> (→"Force":waveform(dbl)[])
    n1446 = Subtract(x=w1441, y="Offset (nm)") -> (x-y=w1618:dbl[])
    n1447 = case shown="True" "Read Lateness and Rel Phase" {
      tunnel: w1461 -> [w1970 w1992]
      tunnel: w1460 -> [w1971 w1991]
      tunnel: [w1970 w1990] -> w1647
      tunnel: [w1971 w1989] -> w1646
      frame False {
      }
      frame True {
        n1448 = xnode "Read/Write Control"("FPGA VI Reference In"=w1992, "error in"=w1991) -> ("FPGA VI Reference Out"=w1990:T18, "error out"=w1989:errorcluster, "GI Relative phase"=→"GI relative phase":i16, "Relative phase"=→"Relative phase (AI1)":i16, "AI Late Counter"=→"Late Counter (AI1)":u16, "GI Late Counter"=→"GI Late Counter":u16, "MCL Late Counter"=→"MCL Late Counter":u16, "MCL Relative Phase"=→"Relative Phase (MCL)":i16, "APD Acq Relative Phase"=→"APD Acq Relative Phase":i16, "APD 1 Gate Relative Phase"=→"APD 1 Gate Relative Phase":i16, "APD 2 Gate Relative Phase"=→"APD 2 Gate Relative Phase":i16, "APD Acq Late Counter"=→"APD Acq Late Counter":u16, "APD 1 Gate Late Counter"=→"APD 1 Gate Late Counter":u16, "APD 2 Gate Late Counter"=→"APD 2 Gate Late Counter":u16, "Green FB Relative Phase"=→"Relative phase (Green FB)":i16, "GI Relative phase 2"=→"GI relative phase 2":i16, "GI Late Counter 2"=→"GI Late Counter 2":u16, "Trap Pos FIFO Timeout"=→"Trap Pos FIFO Timeout":u16, "Trap AI FIFO Timeout"=→"Trap AI FIFO Timeout":u16)
      }
    }
    n1449 = call-poly <vilib>:"Mean.vi"("X"=w1620) -> ("mean"=w1447:dbl)  [unwired: 1 out]
    "T2 X" <- w1447
    n1450 = Negate(x=w1620) -> (-x=w1621:dbl[])
    n1451 = call-poly <vilib>:"Mean.vi"("X"=w1445) -> ("mean"=w1448:dbl)  [unwired: 1 out]
    "T1 X" <- w1448
    n1452 = Negate(x=w1447) -> (-x=w1446:dbl)
    n1453 = Bundle By Name(cluster=w1653, "Y"=w1618) -> (w1592:waveform(dbl))
    "Bead Separation" <- w1592
    n1454 = Add(x=w1445, y=w1621) -> (x+y=w1622:dbl[])
    n1455 = Add(x=w1448, y=w1446) -> (x+y=w1667:dbl)
    n1456 = Subtract(x=w1448, y=w1446) -> (x-y=→"Difference":dbl)
    n1457 = Divide(x=w1622, y=2.0) -> (x/y=→"Vec Mean of T1 T2":dbl[])
    n1458 = Divide(x=w1667, y=2.0) -> (x/y=w1624:dbl)
    "Mean" <- w1624
    n1459 = feedback-in #23("Trap Trig. Fl.") -> ()
    n1460 = feedback #23("Trap Trig. Fl.") -> (w1478:bool)
    n1461 = And(x=w1480, y=w1478) -> (x .and. y?=w1479:bool)
    n1462 = case "If have just turned off triggering" shown="True" w1479 {
      tunnel: w1461 -> [_ w1805]
      tunnel: w1460 -> [_ w1804]
      frame False {
      }
      frame True {
        w1803 = FALSE ("FPGA Trap Trig")
        n1463 = xnode "Read/Write Control"("FPGA VI Reference In"=w1805, "error in"=w1804, "FPGA Trap Trig"=w1803) -> ("FPGA VI Reference Out"=w1802:T18, "error out"=w1801:errorcluster)
        n1464 = xnode "Read/Write Control"("FPGA VI Reference In"=w1802, "error in"=w1801, "TTrig?"=w1803) -> ()  [unwired: 2 out]
        n1465 = local write "Initializing"(FALSE ("Initializing")) -> ()
        n1466 = local write "Triggered"(FALSE ("Triggered")) -> ()
        n1467 = local write "Waiting"(FALSE ("Waiting")) -> ()
      }
    }
    n1468 = Not(x=w1478) -> (.not. x?=w1491:bool)
    n1469 = And(x="Trap Trig. Fl.", y=w1491) -> (x .and. y?=w1488:bool)
    n1470 = local read "Tether"() -> (w1625:bool)
    n1471 = Or(x=w1488, y="Reinitialize") -> (x .or. y?=w1474:bool)
    n1472 = feedback #24(w1484) -> (w1489:string)
    n1473 = Select(t=w1484, s=w1488, f=w1489) -> (s? t:f=w1483:string)
    n1474 = Select(t=w1484, s="Reinitialize", f=w1483) -> (s? t:f=w1482:string)
    n1475 = feedback #25(0) -> (w1486:i32)
    n1476 = feedback #26(w1618) -> (w1617:dbl[])
    n1477 = Build Array (concatenate)(w1618, w1617) -> (w1442:dbl[])
    n1478 = case "For determining if there is a tether still" shown="True" w1625 {
      tunnel: w1624 -> [_ w1929]
      frame False {
      }
      frame True {
        n1479 = Greater?(x="Lost Tether Alarm Threshold (pN)", y=w1929) -> (0:w1927:bool)
        n1480 = case shown="True" w1927 {
          frame False {
          }
          frame True {
            w1930 = FALSE ("Value (Signaling)")
            n1481 = flat-sequence {
              frame #0 {
                # "stop only if saving"
                n1482 = local read "Saving..."() -> (w1942:bool)
                n1483 = And(x=w1942, y="TA Cancel Save?") -> (x .and. y?=w1941:bool)
                n1484 = local write "Stop Saving"(w1941) -> ()
              }
              frame #1 {
                n1485 = case shown="True" "TA Green Off?" {
                  frame False {
                  }
                  frame True {
                    w1945 = FALSE ("Fl. Triggered...")
                    n1486 = local write "Fl. Triggered..."(w1945) -> ()
                    n1487 = property on="Green Laser ON/Interlacing" class="Bool (strict)"("Val(Sgnl)"=w1945) -> ()  [unwired: 2 in, 2 out]
                  }
                }
              }
            }
            n1488 = local read "Time tether formed"() -> (w1936:timestamp)
            n1489 = Get Date/Time In Seconds() -> (seconds since 1Jan1904=w1937:timestamp)
            n1490 = Subtract(x=w1937, y=w1936) -> (x-y=w1935:dbl)
            n1491 = Number To Decimal String(number=w1935) -> (decimal integer string=w1932:string)  [unwired: 1 out]
            n1492 = local read "Messages"() -> (w1939:string)
            n1493 = call <vilib>:"Beep.vi"() -> ()  [unwired: 3 in, 9 out]
            n1494 = Concatenate Strings("Lost tether (" ("Message to add"), w1932, " s)." ("string")) -> (w1934:string)
            n1495 = local write "Tether"(FALSE ("Tether")) -> ()
            n1496 = call "Update messages.vi"("Message to add"=w1934, "Old message string"=w1939) -> ("New message string"=w1938:string)
            n1497 = local write "Messages"(w1938) -> ()
            n1498 = property on="Fl. Triggered..." class="Bool (strict)"("Val(Sgnl)"=w1930) -> ()  [unwired: 2 in, 2 out]
            n1499 = local write "Dip for Protein"(w1930) -> ()
            n1500 = property on="Trap Pos. FB ON" class="Bool (strict)"("Val(Sgnl)"=w1930) -> ()  [unwired: 2 in, 2 out]
            n1501 = property on="Trap Trig. Fl." class="Bool (strict)"("Val(Sgnl)"=w1930) -> ()  [unwired: 2 in, 2 out]
          }
        }
      }
    }
    n1502 = case "For triggering actions based on the trap position (e.g., turning the excitation laser on if trap under feedback moves so far)" shown="True" "Trap Trig. Fl." {
      tunnel: w1469 -> [_ w1818]
      tunnel: w1482 -> [_ w1817]
      tunnel: ["" ("t") w1816] -> w1490
      tunnel: w1474 -> [_ w1815]
      tunnel: [0 ("t") w1814] -> w1487
      tunnel: w1486 -> [_ w1813]
      tunnel: w1461 -> [_ w1812]
      tunnel: w1460 -> [_ w1811]
      frame False {
      }
      frame True {
        n1503 = case shown="\"Wait for trigger\"" w1817 {
          tunnel: w1818 -> [w1835 _ _ w1883]
          tunnel: [w1832 w1864 "" ("t") w1886] -> w1816
          tunnel: w1815 -> [_ _ _ w1874]
          tunnel: [w1831 w1861 0 ("t") w1875] -> w1814
          tunnel: w1813 -> [_ w1863 _ w1881]
          tunnel: w1812 -> [w1820 w1858 _ w1877]
          tunnel: w1811 -> [w1819 w1857 _ w1876]
          frame "Wait for trigger" {
            n1504 = local read "Trap Trig. (FPGA)"() -> (w1823:bool)
            n1505 = Subtract(x=w1835, y="Mean T1 Position\nto compare (nm)") -> (x-y=w1828:dbl[])
            n1506 = call <vilib>:"Std Deviation and Variance.vi"("X"=w1828) -> ("mean"=→"mean":dbl, "standard deviation"=→"standard\ndeviation":dbl)  [unwired: 1 in, 1 out]
            n1507 = Array Max & Min(array=w1828) -> (max value=→"max value":dbl, min value=→"min value":dbl)  [unwired: 2 out]
            n1508 = Greater?(x=w1828, y="Threshold (nm)") -> (0:w1838:bool[])
            n1509 = case shown="True" w1823 {
              tunnel: w1820 -> [_ w1844]
              tunnel: w1819 -> [_ w1843]
              tunnel: [FALSE ("TTrig?") w1842] -> w1826
              frame False {
              }
              frame True {
                n1510 = xnode "Read/Write Control"("FPGA VI Reference In"=w1844, "error in"=w1843) -> ("TTrig?"=w1842:bool)  [unwired: 2 out]
              }
            }
            n1511 = Or Array Elements(Boolean array=w1838) -> (logical OR=w1825:bool)
            n1512 = Select(t=w1826, s=w1823, f=w1825) -> (s? t:f=w1824:bool)
            n1513 = Not(x=w1823) -> (.not. x?=w1822:bool)
            n1514 = And(x=w1824, y=w1822) -> (x .and. y?=w1821:bool)
            n1515 = Select(t="Triggered", s=w1824, f="Wait for trigger") -> (s? t:f=w1832:string)
            n1516 = case shown="True" w1824 {
              tunnel: [0 0] -> w1831
              tunnel: w1820 -> [_ w1849]
              tunnel: w1819 -> [_ w1848]
              frame False {
                "Waiting" <- TRUE ("Waiting")
              }
              frame True {
                n1517 = xnode "Read/Write Control"("FPGA VI Reference In"=w1849, "error in"=w1848, "TTrig?"=FALSE) -> ()  [unwired: 2 out]
                n1518 = local read "Messages"() -> (w1852:string)
                n1519 = call <vilib>:"Beep.vi"() -> ()  [unwired: 12 in]
                n1520 = call "Update messages.vi"("Message to add"="Unwinding trigger.", "Old message string"=w1852) -> ("New message string"=w1853:string)
                n1521 = local write "Messages"(w1853) -> ()
                n1522 = local write "Waiting"(FALSE ("Waiting")) -> ()
                "Triggered" <- TRUE ("Triggered")
              }
            }
            n1523 = case "Only need to turn on laser if host triggered" shown="True" w1821 {
              frame False {
              }
              frame True {
                n1524 = property on="Green Laser ON/Interlacing" class="Bool (strict)"("Val(Sgnl)"=TRUE ("Value (Signaling)")) -> ()  [unwired: 2 in, 2 out]
              }
            }
          }
          frame "Triggered" {
            n1525 = local read "Trap Trig. (FPGA)"() -> (w1860:bool)
            n1526 = Increment(x=w1863) -> (x+1=w1861:i32)
            n1527 = Greater Or Equal?(x=w1861, y="Fl. ON time (n)") -> (x >= y?=w1859:bool)
            n1528 = Select(t="Wait for trigger", s=w1859, f="Triggered" ("t")) -> (s? t:f=w1864:string)
            n1529 = And(x=w1859, y=w1860) -> (x .and. y?=w1856:bool)
            n1530 = case shown="True" w1856 {
              tunnel: w1858 -> [_ w1868]
              tunnel: w1857 -> [_ w1867]
              frame False {
              }
              frame True {
                n1531 = xnode "Read/Write Control"("FPGA VI Reference In"=w1868, "error in"=w1867, "FPGA Trap Trig"=TRUE) -> ()  [unwired: 2 out]
              }
            }
            n1532 = case shown="True" w1859 {
              frame False {
              }
              frame True {
                w1870 = FALSE ("Value (Signaling)")
                n1533 = local write "Triggered"(w1870) -> ()
                n1534 = local write "Waiting"(TRUE ("Waiting")) -> ()
                n1535 = property on="Green Laser ON/Interlacing" class="Bool (strict)"("Val(Sgnl)"=w1870) -> ()  [unwired: 2 in, 2 out]
              }
            }
          }
          frame "Do nothing" {
          }
          frame "Initialize", Default {
            n1536 = Increment(x=w1881) -> (x+1=w1885:i32)
            n1537 = Select(t=1, s=w1874, f=w1885) -> (s? t:f=w1875:i32)
            n1538 = feedback #27(w1883) -> (w1889:dbl[])
            n1539 = Build Array (concatenate)(w1883, w1889) -> (w1882:dbl[])
            n1540 = Greater Or Equal?(x=w1875, y="Wait to get offset (n)") -> (x >= y?=w1878:bool)
            n1541 = Select(t=w1883, s=w1874, f=w1882) -> (s? t:f=w1884:dbl[])
            n1542 = feedback-in #27(w1884) -> ()
            n1543 = call-poly <vilib>:"Mean.vi"("X"=w1884) -> ("mean"=w1879:dbl)  [unwired: 1 out]
            n1544 = local write "Mean T1 Position\nto compare (nm)"(w1879) -> ()
            n1545 = case shown="True" w1874 {
              tunnel: w1877 -> [_ w1895]
              tunnel: w1876 -> [_ w1894]
              frame False {
              }
              frame True {
                w1891 = FALSE ("FPGA Trap Trig")
                n1546 = xnode "Read/Write Control"("FPGA VI Reference In"=w1895, "error in"=w1894, "FPGA Trap Trig"=w1891) -> ("FPGA VI Reference Out"=w1893:T18, "error out"=w1892:errorcluster)
                n1547 = xnode "Read/Write Control"("FPGA VI Reference In"=w1893, "error in"=w1892, "TTrig?"=w1891) -> ()  [unwired: 2 out]
              }
            }
            n1548 = Select(t="Wait for trigger", s=w1878, f="Initialize") -> (s? t:f=w1886:string)
            n1549 = case shown="True" w1878 {
              tunnel: w1879 -> [_ w1898]
              tunnel: w1877 -> [_ w1907]
              tunnel: w1876 -> [_ w1906]
              frame False {
                n1550 = local write "Waiting"(FALSE ("Waiting")) -> ()
                "Initializing" <- TRUE ("Initializing")
              }
              frame True {
                n1551 = local read "Threshold (nm)"() -> (w1910:dbl)
                n1552 = local read "AOM X Cal (nm/MHz)"() -> (w1909:dbl)
                n1553 = Add(x=w1898, y=w1910) -> (x+y=w1911:dbl)
                n1554 = Divide(x=w1911, y=w1909) -> (x/y=w1908:dbl)
                n1555 = call "IR AOM freq to word.vi"("Frequency In (MHz)"=w1908) -> ("Frequency Word Out (double)"=w1905:dbl)
                n1556 = local write "Initializing"(FALSE ("Initializing")) -> ()
                n1557 = local write "Waiting"(TRUE ("Waiting")) -> ()
                n1558 = To Quad Integer(1:w1905) -> (0:w1904:i64)
                n1559 = xnode "Read/Write Control"("FPGA VI Reference In"=w1907, "error in"=w1906, "FPGA TTrig Thresh"=w1904) -> ("FPGA VI Reference Out"=w1901:T18, "error out"=w1900:errorcluster)
                n1560 = xnode "Read/Write Control"("FPGA VI Reference In"=w1901, "error in"=w1900, "FPGA Trap Trig"=TRUE) -> ()  [unwired: 2 out]
              }
            }
          }
        }
      }
    }
    n1561 = feedback-in #24(w1490) -> ()
    n1562 = feedback-in #25(w1487) -> ()
    n1563 = Split 1D Array(array=w1442, index=w1504) -> (first subarray=w1614:dbl[])  [unwired: 1 out]
    n1564 = feedback-in #26(w1614) -> ()
    n1565 = call-poly <vilib>:"Mean.vi"("X"=w1614) -> ("mean"=w1613:dbl)  [unwired: 1 out]
    "Bead Mean (nm)" <- w1613
    n1566 = Subtract(x=w1614, y=w1613) -> (x-y=w1612:dbl[])
    n1567 = Square(x=w1612) -> (x^2=w1611:dbl[])
    n1568 = call-poly <vilib>:"Mean.vi"("X"=w1611) -> ("mean"=w1610:dbl)  [unwired: 1 out]
    n1569 = Square Root(x=w1610) -> (sqrt(x)=w1609:dbl)
    n1570 = Multiply(x=10.0, y=w1609) -> (x*y=→"RMS (Ang)":dbl)
    n1571 = xnode ("Read/Write Control")("FPGA VI Reference In"=w1647, "error in"=w1646) -> ("FPGA VI Reference Out"=w1472:T18, "error out"=w1471:errorcluster, "AI2 Y Sum Set 1"=w1745:i16, "AI2 Y Sum Set 2"=w1744:i16, "AI1 X Set 1"=w1536:fxp<+/-,16,1>, "AI1 X Set 2"=w1535:fxp<+/-,16,1>, "Trap Pos FB Int Signal"=→"Trap Pos FB Int Signal":fxp<+/-,24,9>, "Trap Pos FB Int-Norm Signal"=→"Trap Pos FB Int-Norm Signal":fxp<+/-,16,1>, "Trap Pos FB Action"=w1529:i64, "Scanning"=→"AOD Scanning":bool, "Scan I"=→"AOD Scan I":u64, "Scanning MCL"=w1747:bool, "Scan I (MCL)"=→"MCL Scan I":u64, "Green FB Sum"=w1684:i16, "Trap Pos FB Action"=w1459:i64, "TTrig Fin Thresh"=w1455:i64)
    "MCL Scanning" <- w1747
    "Trap Pos FB Action" <- w1529
    n1572 = local read "FB Trig Integrate"() -> (w1453:u32)
    n1573 = Divide(x=w1684, y=3276.7) -> (x/y=→"Green laser plot" →"Green laser intensity (V)":dbl)
    n1574 = Divide(x=w1459, y=w1453) -> (x/y=w1452:dbl)
    "TTrig Sig (Int)" <- w1452
    n1575 = Divide(x=w1455, y=w1453) -> (x/y=w1450:dbl)
    "TTrig Fin Thresh (Int)" <- w1450
    n1576 = local read "AOM X Cal (nm/MHz)"() -> (w1458:dbl)
    n1577 = local read "AI2 (V)"() -> (w1746:cluster{"Set 1":dbl, "Set 2":dbl})
    n1578 = Bundle By Name(cluster=w1746, "Set 1"=w1745, "Set 2"=w1744) -> (w1742:cluster{"Set 1":dbl, "Set 2":dbl})
    n1579 = Divide(x=w1529, y=327.67) -> (x/y=→"Action (%)":dbl)
    n1580 = local read "Trap X (AI1)"() -> (w1549:T10)
    n1581 = call "IR AOM word double to freq.vi"("Frequency Word In (double)"=w1450) -> ("Frequency Out (MHz)"=w1449:dbl)
    n1582 = call "IR AOM word double to freq.vi"("Frequency Word In (double)"=w1452) -> ("Frequency Out (MHz)"=w1451:dbl)
    n1583 = Divide(x=w1742, y=3276.7) -> (x/y=w1741:cluster{"Set 1":dbl, "Set 2":dbl})
    n1584 = Multiply(x=w1451, y=w1458) -> (x*y=w1457:dbl)
    "TTrig Sig (nm)" <- w1457
    n1585 = Multiply(x=w1449, y=w1458) -> (x*y=w1456:dbl)
    "TTrig Fin Thresh (nm)" <- w1456
    n1586 = local write "AI2 (V)"(w1741) -> ()
    n1587 = Bundle(cluster=w1549, "Trap 1"=w1536, "Trap 2"=w1535) -> (→"Trap X (AI1)":T10)
    n1588 = Bundle(w1457, w1456) -> (→"TTrig":cluster{dbl, dbl})  [unwired: 1 in]
    n1589 = flat-sequence "To save data" {
      tunnel: [w2766] -> w1765
      tunnel: [w2767] -> w1764
      tunnel: w1715 -> [w2760]
      tunnel: w1477 -> [w2764]
      tunnel: ["Save Calibration"] -> w1738
      tunnel: w1735 -> [w2763]
      tunnel: [w2756] -> w1734
      tunnel: [w2753] -> w1733
      tunnel: [w2750] -> w1732
      tunnel: w1714 -> [w2752]
      tunnel: w1629 -> [w2746]
      tunnel: [w2746] -> w1628
      tunnel: ["Start Saving"] -> w1594
      tunnel: [w2740] -> w1517
      tunnel: [w2739] -> w1516
      tunnel: w1765 -> [w3002]
      tunnel: w1764 -> [w3001]
      tunnel: w1518 -> [w3000]
      tunnel: w1738 -> [w2999]
      tunnel: w1734 -> [w2997]
      tunnel: w1733 -> [w2996]
      tunnel: w1732 -> [w2995]
      tunnel: w1603 -> [w2994]
      tunnel: w1639 -> [w2993]
      tunnel: w1628 -> [w2992]
      tunnel: w1594 -> [w2991]
      tunnel: w1592 -> [w2990]
      tunnel: w1568 -> [w2989]
      tunnel: w1517 -> [w2988]
      tunnel: w1516 -> [w2987]
      tunnel: w1515 -> [w2986]
      tunnel: w1438 -> [w2985]
      frame #0 {
        n1590 = Or(x="Save N Sets", y="Start Saving") -> (x .or. y?=w2747:bool)
        n1591 = To Double Precision Float(number=w2763) -> (double precision float=w2757:dbl)
        n1592 = Build Array(w2747, "Save Calibration", w2760, w2752) -> (w2762:bool[])
        n1593 = Compound Arithmetic op=OR("Save Calibration", w2760, w2747, w2752) -> (w2765:bool)
        n1594 = Boolean Array To Number(Boolean array=w2762) -> (number=w2759:u32)
        n1595 = feedback #28(FALSE ("Save APD Data\nwith Trap Data")) -> (w2741:bool)
        n1596 = feedback #29(refnum<k0> refnum) -> (w2768:refnum<file>)
